vi "xeva-setTime.vi"(3 "error in (no error)":errorcluster, 4 "xeva-time":dbl, 5 "xeva-camref":T1) -> (0 "error out":errorcluster, 1 "xeva-time-ok":bool)   [LabVIEW 2017]
uses:
  <vilib>/Xenics Infrared Solutions/Xeneth LabVIEW API/VIs/Controls/Camara.ctl
  <vilib>/Xenics Infrared Solutions/Xeneth LabVIEW API/VIs/Property/XC Set Property Value L.vi
  <vilib>/Xenics Infrared Solutions/Xeneth LabVIEW API/Xeneth.lvlib
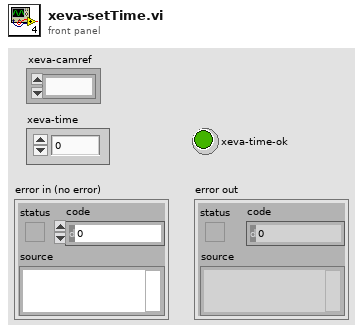
[diagram p1: front panel]
types:
  T1 = typedef "Xeneth.lvlib/Camara.ctl" = refnum<k1>
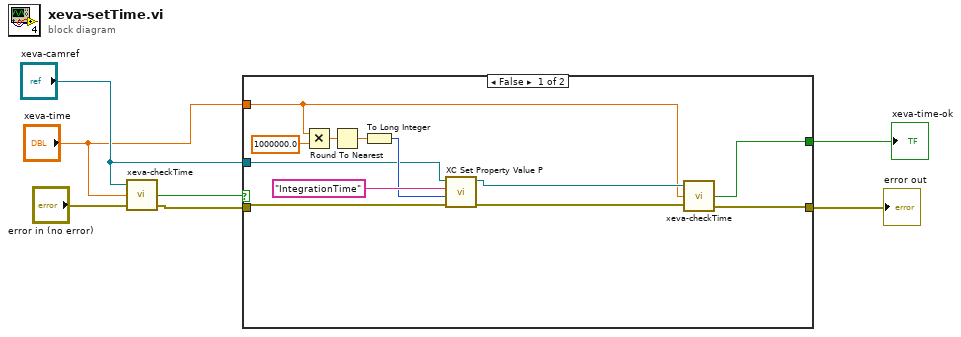
[diagram p0: block diagram]
diagram:
  n1 = call "xeva-checkTime.vi"("error in (no error)"="error in (no error)", "xeva-time"="xeva-time", "xeva-camref"="xeva-camref") -> ("error out"=w5:errorcluster, "xeva-time-ok"=w6:bool)  [unwired: 1 in]
  n2 = case shown="False" w6 {
    selector: w6 -> [_ w20]
    tunnel: [w9 w21] -> w4
    tunnel: w5 -> [w18 w21]
    tunnel: "xeva-camref" -> [w14 _]
    tunnel: "xeva-time" -> [w10 _]
    tunnel: [w8 w20] -> w1
    frame False {
      n3 = Multiply(x=w10, y=1000000.0 ("x")) -> (x*y=w17:dbl)
      n4 = Round To Nearest(number=w17) -> (nearest integer value=w16:dbl)
      n5 = To Long Integer(number=w16) -> (32bit integer=w15:i32)
      n6 = call-poly <vilib>:"XC Set Property Value P.vi"("error in (no error)"=w18, "lValue"=w15, "pPrp"="IntegrationTime", "Cam Ref"=w14) -> ("error out"=w12:errorcluster, "Cam Ref Out"=w13:T1)  [unwired: 6 in]
      n7 = call "xeva-checkTime.vi"("error in (no error)"=w12, "xeva-time"=w10, "xeva-camref"=w13) -> ("error out"=w9:errorcluster, "xeva-time-ok"=w8:bool)  [unwired: 1 in]
    }
    frame True {
    }
  }
  "error out" <- w4
  "xeva-time-ok" <- w1
